vi "niFpgaZero-OrderHoldTemplate.vi"(0 "input":fxp<+/-,16,16>, 1 "reset":bool, 7 "hold time in cycles":u16) -> (4 "output":fxp<+/-,16,16>)   [LabVIEW 2017]
doc: "Samples an input signal and holds it for a specified number of calls to the VI. The data type you wire to <B>input</B> determines the <B>output</B> data type."
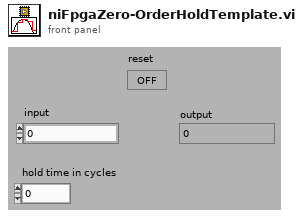
[diagram p1: front panel]
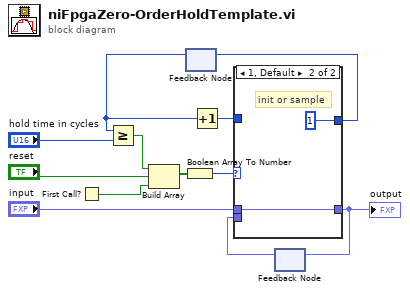
[diagram p0: block diagram]
diagram:
  n1 = First Call?() -> (First Call?: T/F=w11:bool)
  n2 = feedback #1() -> (w6:u16)  [unwired: 1 in]
  n3 = Greater Or Equal?(x=w6, y="hold time in cycles") -> (x >= y?=w9:bool)
  n4 = Build Array(w9, "reset", w11) -> (w8:bool[])
  n5 = Boolean Array To Number(Boolean array=w8) -> (number=w7:u8)
  n6 = Increment(x=w6) -> (x+1=w5:u16)
  n7 = feedback #2() -> (w4:fxp<+/-,16,16>)  [unwired: 1 in]
  n8 = case shown="1, Default" w7 {
    tunnel: [w13 u16 1] -> w12
    tunnel: [w14 w15] -> w1
    tunnel: w4 -> [w14 _]
    tunnel: w5 -> [w13 _]
    tunnel: "input" -> [_ w15]
    frame 0 {
      # "holding"
    }
    frame 1, Default {
      # "init or sample"
    }
  }
  "output" <- w1
  n9 = feedback-in #1(w12) -> ()
  n10 = feedback-in #2(w1) -> ()
